vi "控制曲线是否可见（图例与属性）.vi"() -> ()   [LabVIEW 2012]
uses:
  <vilib>/Analysis/NI_AALBase.lvlib
panel:
  out "Waveform Graph":dbl[][](graph)
  in  "Active":bool[](array[boolean])
  in  "stop":bool
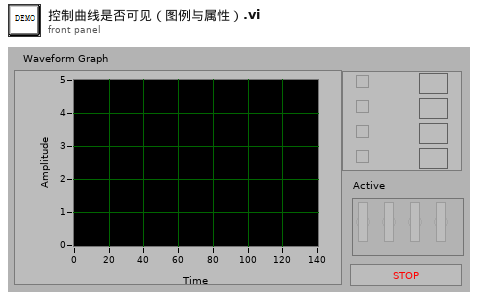
[diagram p1: front panel]
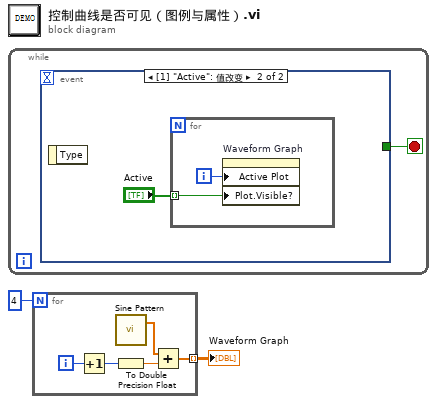
[diagram p0: block diagram]
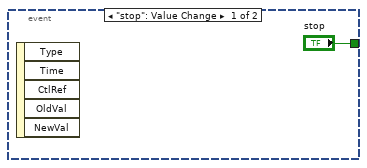
[diagram p2: hidden frame]
diagram:
  n1 = while {
    stop <- w3 stop-if-true
    n2 = event shown="[1] \"Active\": 值改变" {
      selector: _ -> [_ _]
      dyn-events: _ -> [_ _]
      timeout: _ -> [_ _]
      tunnel: ["stop" _] -> w3
      event "stop": Value Change {
        n3 = event-data() -> ()  [unwired: 1 in, 5 out]
      }
      event "Active": Value Change {
        n4 = event-data() -> ()  [unwired: 1 in, 1 out]
        n5 = for {
          tunnel: "Active" -> [w6] mode=indexing
          i -> [w7]
          n6 = property on="Waveform Graph" class="WFGraph (严格)"("Active Plot"=w7, "Plot.Visible?"=w6) -> ()  [unwired: 2 in, 2 out]
        }
      }
    }
  }
  n7 = for {
    N: 4 -> [_]
    tunnel: [w8] -> w1 mode=indexing
    i -> [w12]
    n8 = Increment(x=w12) -> (x+1=w11:i32)
    n9 = call <vilib>:"Sine Pattern.vi"() -> ("Sinusoidal Pattern"=w10:dbl[])  [unwired: 4 in, 1 out]
    n10 = To Double Precision Float(number=w11) -> (double precision float=w9:dbl)
    n11 = Add(x=w10, y=w9) -> (x+y=w8:dbl[])
  }
  "Waveform Graph" <- w1
